vi "Simple Read Lock-in DAQ - One board.vi"(4 "Lock-in settings":T1={"Sine Frequency, Hz"=0.0, "Time constant, s"=0.12500000000000006, "Low-pass filter"=enum."Butterworth", "Output representation"=enum."Real/Imaginary", "Phases, deg"=[], "Low-pass filter Order"=1, "Decimating factor"=1, "Samples to Read"=10000, "Post-filter decimation"=1, "Blocks to average"=1, "Trig delay, points"=0, "Harmonics per channel"=[], "Amplitude scale"=enum."Amplitude"} {"Time constant, s" format="%.1e"}, 6 "Initialize?":bool, 7 "Amplitude scale":enum16{"Amplitude", "RMS", "Peak-to-Peak"}(ring)=enum."RMS", 8 "error in (no error)":errorcluster, 9 "DAQ timeout, s":dbl=10.0 format="%0.2f", 11 "DAQ task":refnum<k21>) -> (0 "error out":errorcluster, 1 "Avg. signal Array":dbl[](array[numeric]), 2 "signal(s) out (DBL)":dbl[][](array[numeric]), 3 "DAQ task out":refnum<k21>, 5 "signal(s) out (WFM)":waveform(dbl)[](array[waveform]))   [LabVIEW 2020]
uses:
  <vilib>/Waveform/WDTOps.llb/WDT Append Waveforms DBL.vi
  <vilib>/Waveform/WDTOps.llb/WDT Number of Waveform Samples DBL.vi
  Lockin Settings.ctl
  Harmonics per channel.ctl
panel:
  out "Waveform Graph 2":dbl[](graph)
  out "number of samples":i32
  out "Waveform Graph":waveform(dbl)[](graph)
  out "AvailSampPerChan":u32
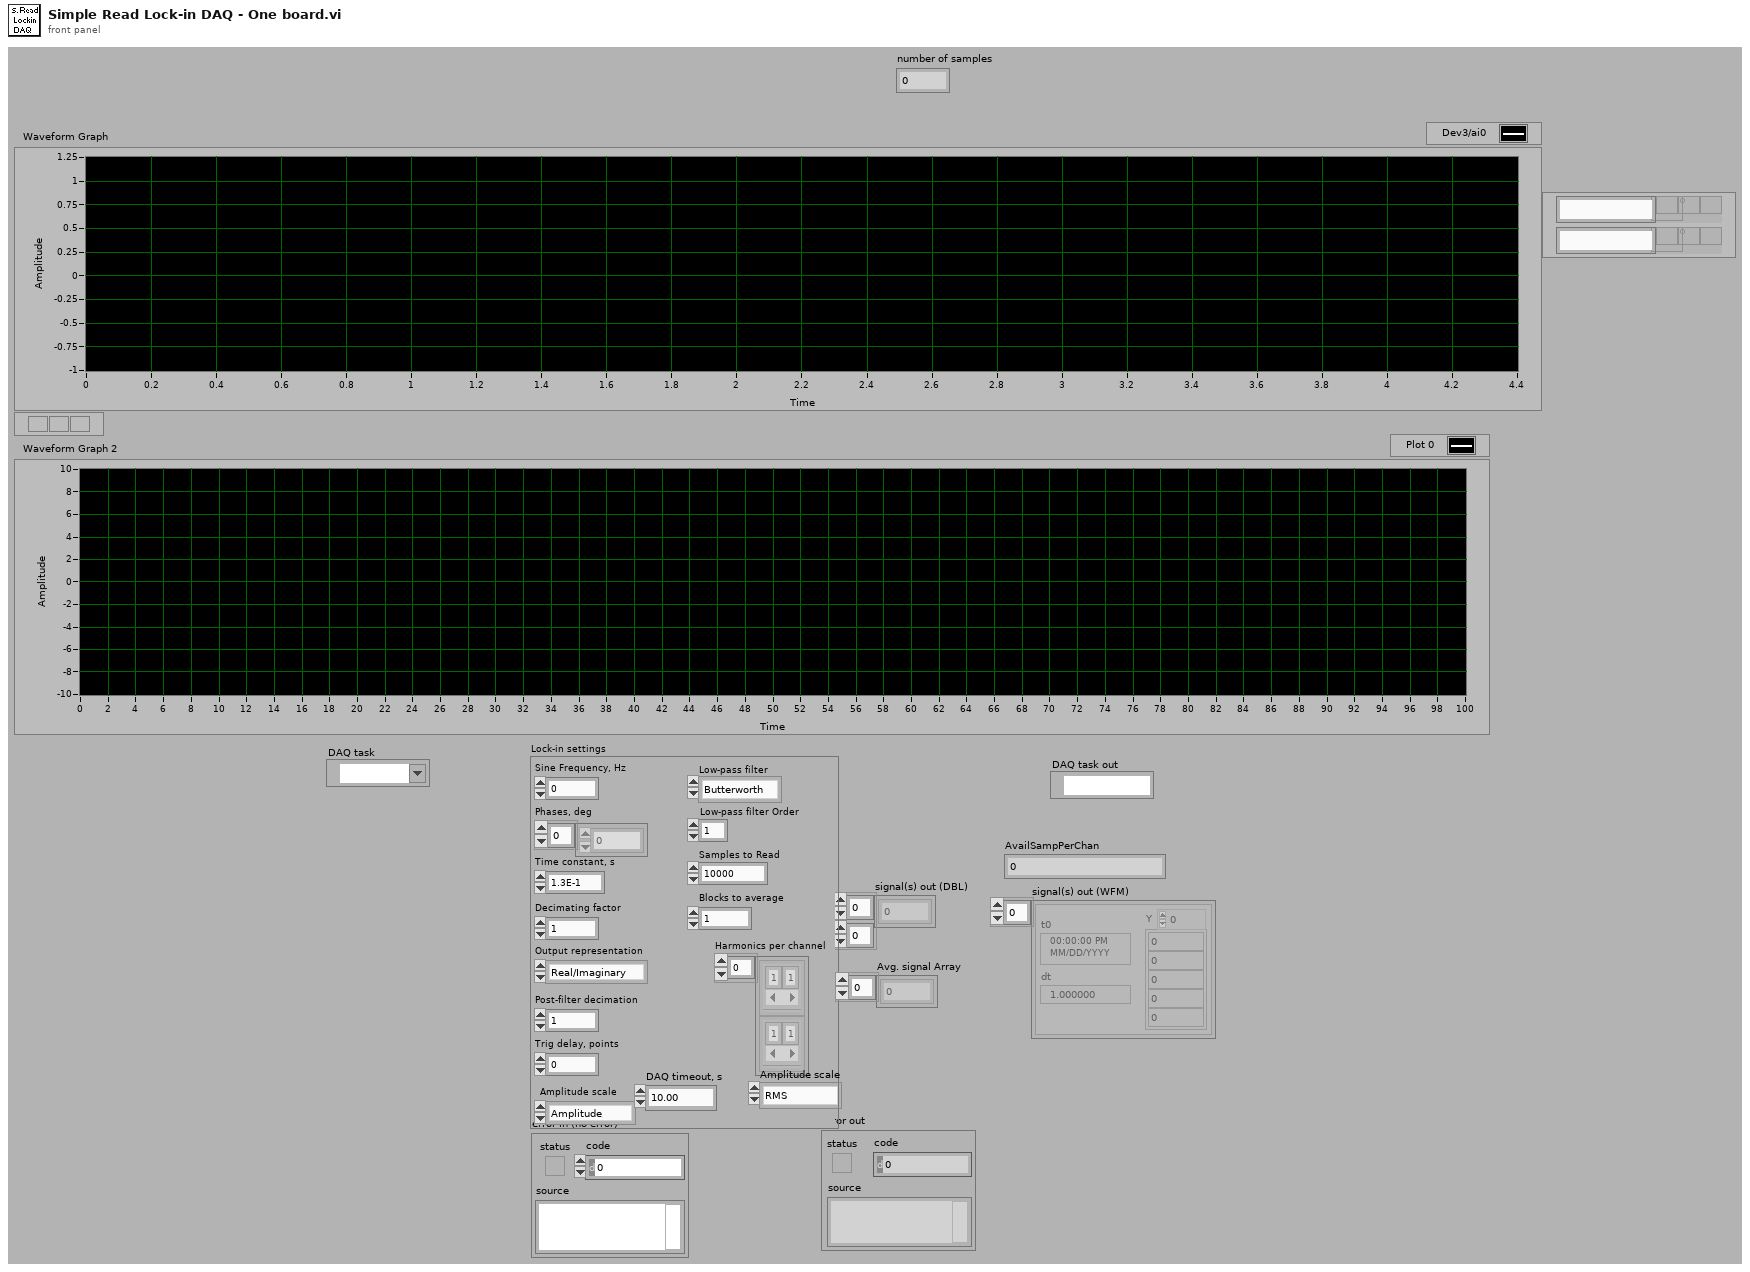
[diagram p1: front panel]
types:
  T1 = typedef "Lockin Settings.ctl" = cluster{"Sine Frequency, Hz":dbl, "Time constant, s":dbl, "Low-pass filter":enum16{"No filtering", "Butterworth", "Bessel"}, "Output representation":enum16{"Real/Imaginary", "Polar"}, "Phases, deg":dbl[], "Low-pass filter Order":i32, "Decimating factor":i32, "Samples to Read":i32, "Post-filter decimation":i32, "Blocks to average":i32, "Trig delay, points":i32, "Harmonics per channel":T2, "Amplitude scale":enum16{"Amplitude", "RMS", "Peak-to-Peak"}}
  T2 = typedef "Harmonics per channel.ctl" = cluster{"Harmonics":i32[]}[]
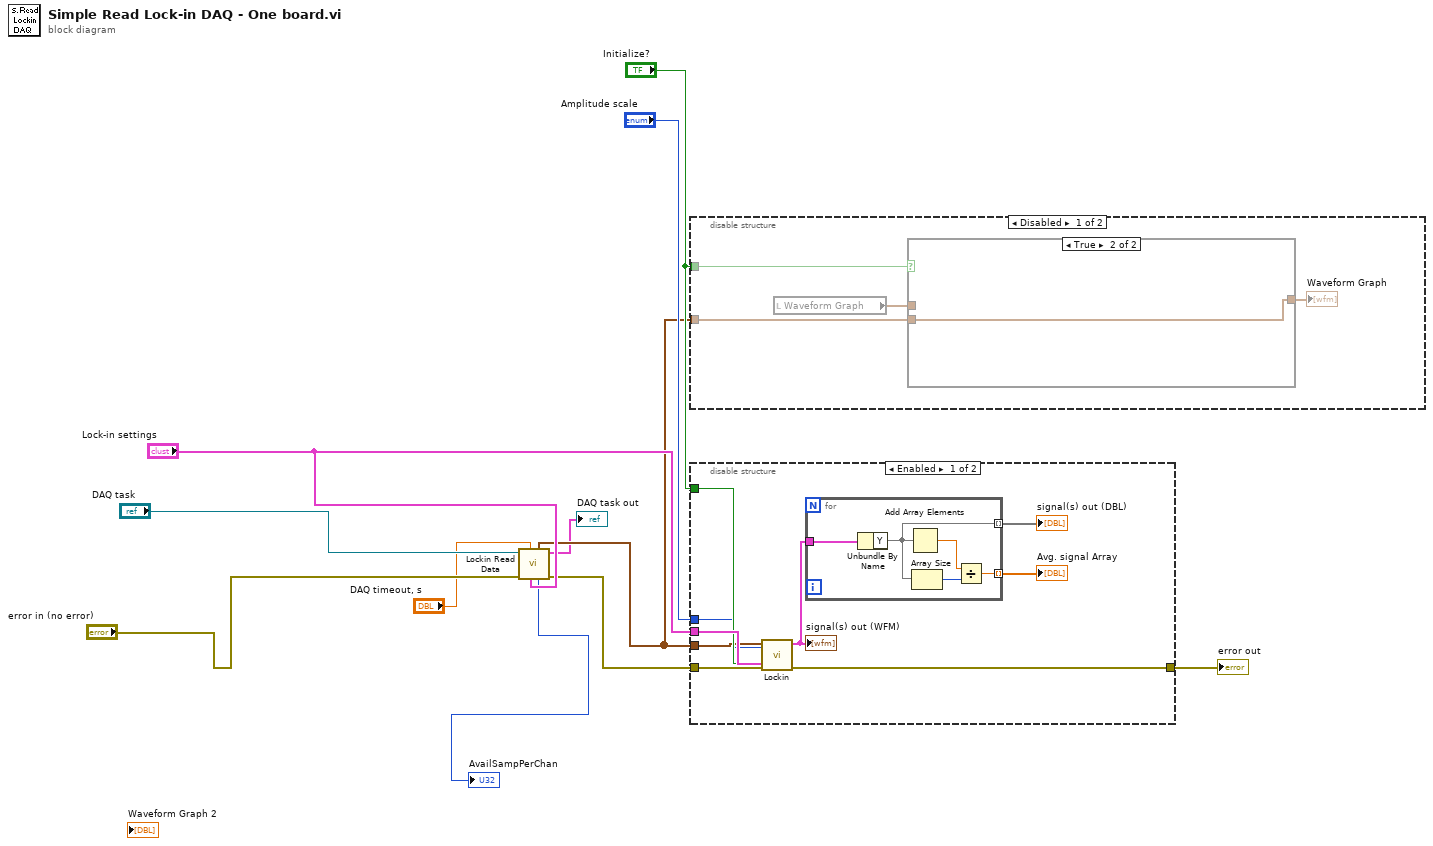
[diagram p0: block diagram]
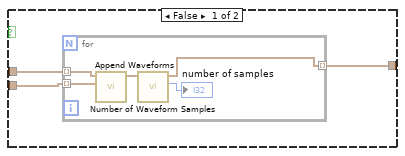
[diagram p2: hidden frame]
diagram:
  n1 = call "Lockin Read Data.vi"(6:"Lock-in settings", "DAQ timeout, s"="DAQ timeout, s", "error in (no error)"="error in (no error)", "Lock-in settings"="DAQ task") -> ("error out"=w2:errorcluster, "Lock-in settings out"=→"DAQ task out":T1, "AvailSampPerChan"=→"AvailSampPerChan":u32, "data"=w4:waveform(dbl)[])  [unwired: 3 in, 1 out]
  n2 = disable-structure shown="Disabled" {
    disable-tunnel: w4 -> [w14 _]
    disable-tunnel: "Initialize?" -> [w12 _]
    frame Disabled {
      n3 = local read "Waveform Graph"() -> (w15:waveform(dbl)[])
      n4 = case shown="True" w12 {
        tunnel: w15 -> [w18 _]
        tunnel: w14 -> [w17 w24]
        tunnel: [w16 w24] -> w13
        frame False {
          n5 = for {
            tunnel: w18 -> [w23] mode=indexing
            tunnel: w17 -> [w22] mode=indexing
            tunnel: [w20] -> w16 mode=indexing
            n6 = call-poly <vilib>:"Append Waveforms.vi"("waveform B"=w22, "waveform A"=w23) -> ("waveform out"=w21:waveform(dbl))  [unwired: 8 in, 1 out]
            n7 = call-poly <vilib>:"Number of Waveform Samples.vi"("waveform in"=w21) -> ("number of samples"=→"number of samples":i32, "waveform out"=w20:waveform(dbl))  [unwired: 8 in, 1 out]
          }
        }
        frame True {
        }
      }
      "Waveform Graph" <- w13
    }
    frame Enabled {
    }
  }
  n8 = disable-structure shown="Enabled" {
    disable-tunnel: "Lock-in settings" -> [w33 _]
    disable-tunnel: [w31 w39] -> w11
    disable-tunnel: "Initialize?" -> [w30 _]
    disable-tunnel: w2 -> [w28 w39]
    disable-tunnel: w4 -> [w27 _]
    disable-tunnel: "Amplitude scale" -> [w25 _]
    frame Enabled {
      n9 = call "Lockin.vi"(4:w33, 6:w30, "Initialize?"=w25, "error in (no error)"=w28, "Lock-in settings"=w27) -> ("error out"=w31:errorcluster, "Lock-in settings out"=w26:T1)  [unwired: 4 in, 1 out]
      "signal(s) out (WFM)" <- w26
      n10 = for {
        tunnel: w26 -> [w38]
        tunnel: [w35] -> w32 mode=indexing
        tunnel: [w34] -> w29 mode=indexing
        n11 = Unbundle By Name(w38) -> ("Y"=w35)
        n12 = Add Array Elements(numeric array=w35) -> (sum=w37:dbl)
        n13 = Array Size(array=w35) -> (size(s)=w36:i32)
        n14 = Divide(x=w37, y=w36) -> (x/y=w34:dbl)
      }
      "signal(s) out (DBL)" <- w32
      "Avg. signal Array" <- w29
    }
    frame Disabled {
    }
  }
  "error out" <- w11
